vi "CursorPositionChanged.vi"(4 "CursorPos x1":u16, 5 "CursorPos x0":u16, 6 "x-values":dbl[](array[numeric]) format="%.2f", 7 "action":enum16{"Check", "Get", "xval"}(ring)) -> (0 "CursorPos min out":u16, 1 "CursorPos max out":u16, 2 "x-values out":dbl[](array[numeric]) format="%.2f", 3 "cursorpos changed?":bool)   [LabVIEW 2009]
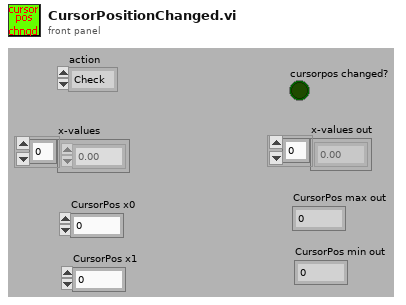
[diagram p1: front panel]
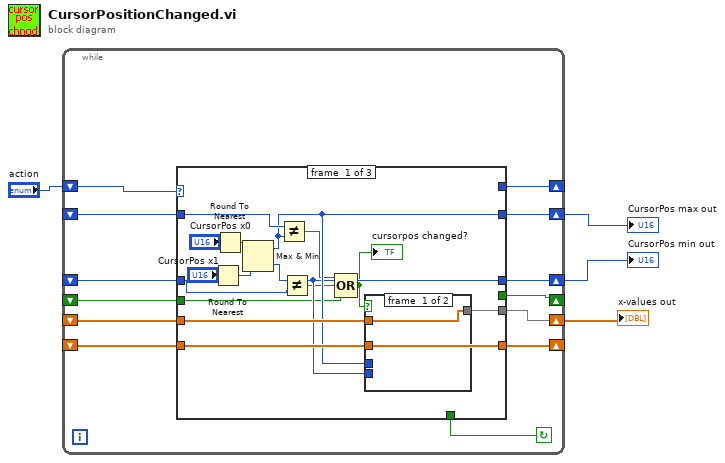
[diagram p0: block diagram]
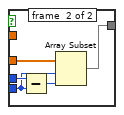
[diagram p2: hidden frame]
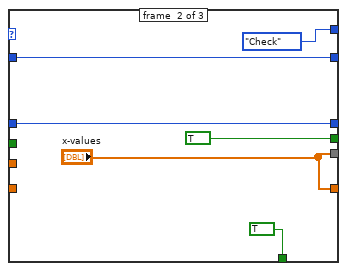
[diagram p3: hidden frame]
diagram:
  n1 = while {
    shift-right: [w17] -> w4
    shift-left: _ -> [w14]
    shift-right: [w16] -> w3
    shift-left: _ -> [w15]
    shift-right: [w13] -> w2
    shift-left: _ -> [w12]
    shift-right: [w9] -> _
    shift-left: "action" -> [w11]
    shift-right: [w8] -> _
    shift-left: _ -> [w7]
    shift-right: [w6] -> _
    shift-left: _ -> [w5]
    stop <- w10 continue-if-true
    n2 = case shown="\"xval\"" w11 {
      tunnel: w14 -> [w29 w42 w48]
      tunnel: [w23 w42 w48] -> w17
      tunnel: [w22 w41 w47] -> w16
      tunnel: w15 -> [w30 w41 w47]
      tunnel: [w26 "x-values" w46] -> w13
      tunnel: w12 -> [w24 _ w46]
      tunnel: [_ TRUE _] -> w10
      tunnel: [_ enum16{"Check", "Get", "xval"}."Check" ("Enum") _] -> w9
      tunnel: [w25 "x-values" w45] -> w8
      tunnel: w7 -> [w25 _ w45]
      tunnel: [_ TRUE _] -> w6
      tunnel: w5 -> [w18 _ _]
      frame #0 {
        n3 = Round To Nearest(number="CursorPos x1") -> (nearest integer value=w28:u16)
        n4 = Round To Nearest(number="CursorPos x0") -> (nearest integer value=w27:u16)
        n5 = Max & Min(x=w27, y=w28) -> (max(x,y)=w23:u16, min(x,y)=w22:u16)
        n6 = Not Equal?(x=w29, y=w23) -> (x != y?=w21:bool)
        n7 = Not Equal?(x=w22, y=w30) -> (x != y?=w20:bool)
        n8 = Compound Arithmetic op=OR(w21, w20, w18) -> (w19:bool)
        "cursorpos changed?" <- w19
        n9 = case shown="False" w19 {
          tunnel: w25 -> [_ w38]
          tunnel: [w33 w37] -> w26
          tunnel: w24 -> [w33 _]
          tunnel: w23 -> [_ w36]
          tunnel: w22 -> [_ w34]
          frame #0 {
          }
          frame #1 {
            n10 = Subtract(x=w36, y=w34) -> (x-y=w35:u16)
            n11 = Array Subset(array=w38, index=w34, length=w35) -> (w37:dbl[])
          }
        }
      }
      frame #1 {
      }
      frame #2 {
      }
    }
  }
  "CursorPos max out" <- w4
  "CursorPos min out" <- w3
  "x-values out" <- w2
